vi "Catch DarkSky Errors.vi"(8 "error in (no error)":errorcluster) -> (0 "error out":errorcluster)   [LabVIEW 2017, in "Dark Sky Weather Data for LabVIEW.lvlib"]
doc: "Checks for possible errors related to entering the parameters needed by the Dark Sky API"
uses:
  Dark Sky Weather Data for LabVIEW.lvlib
  <vilib>/Utility/error.llb/Error Cluster From Error Code.vi
  <vilib>/ErrorRing/Error Ring.xnode
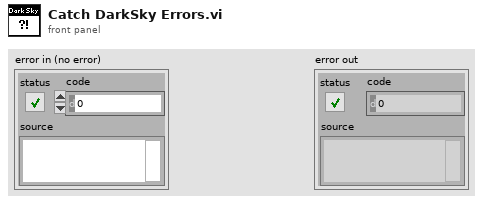
[diagram p1: front panel]
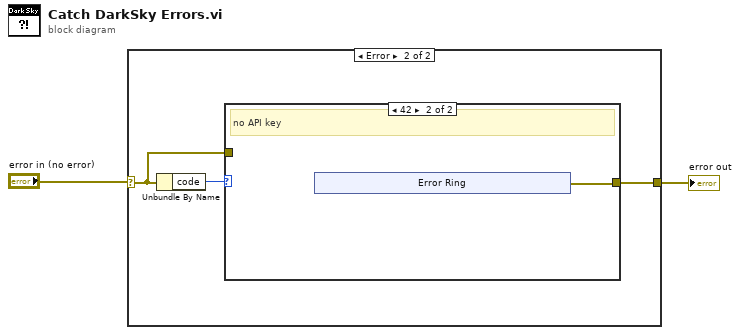
[diagram p0: block diagram]
diagram:
  n1 = case shown="Error" "error in (no error)" {
    selector: "error in (no error)" -> [w3 w5]
    tunnel: [w3 w4] -> w1
    frame No Error {
    }
    frame Error {
      n2 = Unbundle By Name(w5) -> ("code"=w6:i32)
      n3 = case shown="42" w6 {
        tunnel: w5 -> [w7 _]
        tunnel: [w7 w8] -> w4
        frame 0, Default {
          # "Not a Dark Sky-related error"
        }
        frame 42 {
          # "no API key"
          n4 = xnode "Error Ring"() -> ("error out"=w8:errorcluster)
        }
      }
    }
  }
  "error out" <- w1
